vi "GET.vi"(8 "error in (no error)":errorcluster, 9 "parameters":cluster{"name":string, "value":string}[](array[cluster]), 10 "relative URL":string, 11 "eLab in":refnum<class "PL eLabFTW Client.lvclass">) -> (0 "error out":errorcluster, 2 "response body":string, 3 "eLab out":refnum<class "PL eLabFTW Client.lvclass">)   [LabVIEW 2015, in "PL eLabFTW Client.lvclass"]
doc: "Performs GET request with the specified relative URL and parameters and returns the response body."
uses:
  PL eLabFTW Client.lvclass
  PL eLabFTW Client.lvclass/PL eLabFTW Client.ctl
  <vilib>/httpClient/LabVIEWHTTPClient.lvlib
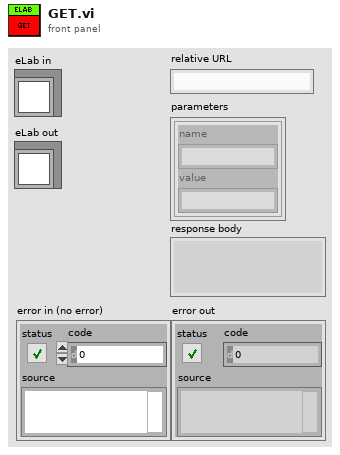
[diagram p1: front panel]
types:
  T1 = typedef "LabVIEWHTTPClient.lvlib/ClientHandle.ctl" = refnum<k1>
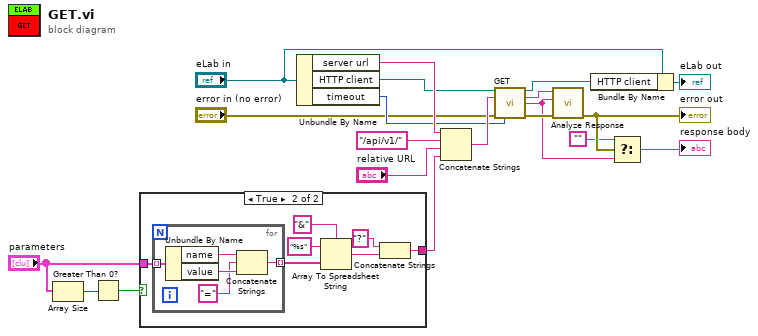
[diagram p0: block diagram]
diagram:
  n1 = Array Size(array="parameters") -> (size(s)=w4:i32)
  n2 = Greater Than 0?(x=w4) -> (x > 0?=w3:bool)
  n3 = case shown="True" w3 {
    tunnel: "parameters" -> [_ w27]
    tunnel: [_ w21] -> w1
    frame False {
    }
    frame True {
      n4 = for {
        tunnel: w27 -> [w32] mode=indexing
        tunnel: [w28] -> w26 mode=indexing
        n5 = Unbundle By Name(w32) -> ("name"=w31:string, "value"=w30:string)
        n6 = Concatenate Strings(w31, "=" ("string"), w30) -> (w28:string)
      }
      n7 = Array To Spreadsheet String(delimiter (Tab)="&", array=w26, 3:"%s" ("format string")) -> (spreadsheet string=w23:string)
      n8 = Concatenate Strings("?" ("string"), w23) -> (w21:string)
    }
  }
  n9 = Unbundle By Name("eLab in") -> ("server url"=w20:string, "HTTP client"=w8:T1, "timeout"=w17:i32)
  n10 = Concatenate Strings(w20, "/api/v1/" ("string"), "relative URL", w1) -> (w18:string)
  n11 = call <vilib>:"GET.vi"("client handle"=w8, "url"=w18, "error in (no error)"="error in (no error)", "timeout (10000)"=w17) -> ("client handle out"=w5:T1, "headers"=w13:string, "body"=w11:string, "error out"=w14:errorcluster)  [unwired: 8 in]
  n12 = call "Analyze Response.vi"("error in (no error)"=w14, "body"=w11, "headers"=w13) -> ("error out"=w12:errorcluster)  [unwired: 8 in]
  "error out" <- w12
  n13 = Bundle By Name(cluster="eLab in", "HTTP client"=w5) -> (→"eLab out":refnum<class "PL eLabFTW Client.lvclass">)
  n14 = Select(t="", s=w12, f=w11) -> (s? t:f=→"response body":string)
